vi "SLSC Create Tree Hierarchy.vi"(7 "Initialized?":bool, 8 "error in (no error)":errorcluster, 9 "SLSC EDS module":T2, 10 "Custom Device Name":string, 11 "Item Ref in":T1 format="%.0x") -> (0 "error out":errorcluster, 3 "Parent Ref out":T1 format="%.0x")   [LabVIEW 2019, in "SLSC EDS System Explorer.lvlib"]
uses:
  System Explorer/SLSC EDS System Explorer.lvlib
  SLSC EDS API/JSON parsing/EDSjsonStructure.ctl
  SLSC EDS API/JSON parsing/enum.ctl
  SLSC EDS API/JSON parsing/property.ctl
  SLSC EDS API/JSON parsing/command.ctl
  SLSC EDS API/JSON parsing/scale.ctl
  SLSC EDS API/JSON parsing/physicalChannel.ctl
  SLSC EDS API/JSON parsing/register.ctl
  <vilib>/NI VeriStand/Custom Device API/Custom Device Item Ref.ctl
  Shared/Constants.vi
  <vilib>/NI VeriStand/Custom Device API/Set Item Property (Boolean).vi
  <vilib>/NI VeriStand/Custom Device API/Set Item Property (Variant).vi
  <vilib>/NI VeriStand/Custom Device API/Set Item Property (U32).vi
  <vilib>/NI VeriStand/Custom Device API/Set Item Property (String).vi
  <vilib>/NI VeriStand/Custom Device API/Get Item Property (U32).vi
  SLSC CD System Explorer.lvlib
  <vilib>/NI VeriStand/Custom Device API/Custom Device API.lvlib
  Shared/SLSC EDS Shared.lvlib
  <vilib>/NI VeriStand/Custom Device Tools/Custom Device Utility Library/Custom Device Utility Library.lvlib
panel:
  # "not working\nregisterMap->registers->initialValue"
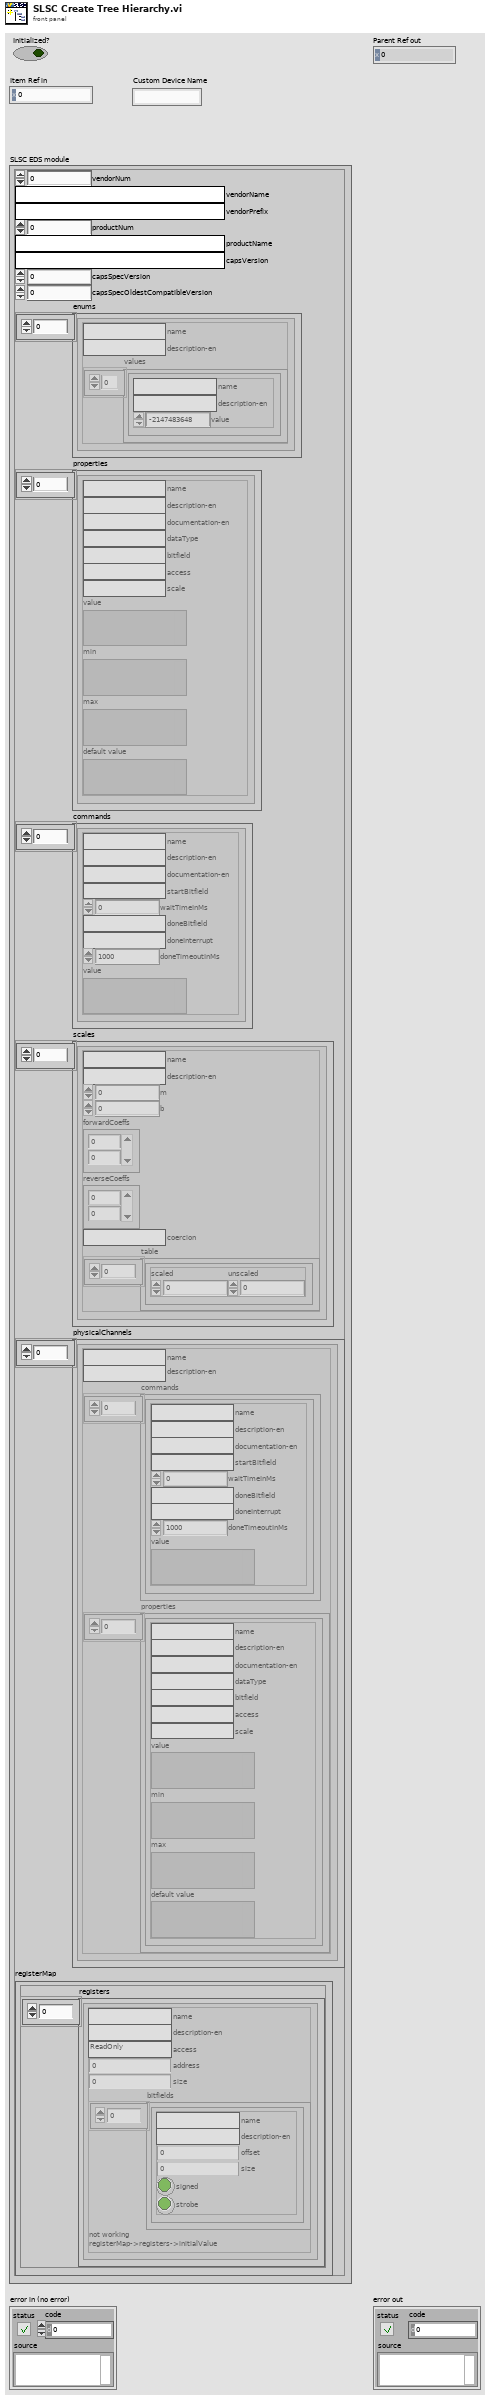
[diagram p1: front panel]
types:
  T1 = typedef "Custom Device API.lvlib/Custom Device Item Ref.ctl" = u64
  T2 = typedef "EDSjsonStructure.ctl" = cluster{"vendorNum":u32, "vendorName":string, "vendorPrefix":string, "productNum":u32, "productName":string, "capsVersion":string, "capsSpecVersion":u32, "capsSpecOldestCompatibleVersion":u32, "enums":T3[], "properties":T4[], "commands":T5[], "scales":T6[], "physicalChannels":T7[], "registerMap":cluster{"registers":T8[]}}
  T3 = typedef "enum.ctl" = cluster{"name":string, "description-en":string, "values":cluster{"name":string, "description-en":string, "value":i32}[]}
  T4 = typedef "property.ctl" = cluster{"name":string, "description-en":string, "documentation-en":string, "dataType":string, "bitfield":string, "access":string, "scale":string, "value":variant, "min":variant, "max":variant, "default value":variant}
  T5 = typedef "command.ctl" = cluster{"name":string, "description-en":string, "documentation-en":string, "startBitfield":string, "waitTimeInMs":i32, "doneBitfield":string, "doneInterrupt":string, "doneTimeoutInMs":i32, "value":variant}
  T6 = typedef "scale.ctl" = cluster{"name":string, "description-en":string, "m":dbl, "b":dbl, "forwardCoeffs":dbl[], "reverseCoeffs":dbl[], "coercion":string, "table":cluster{"scaled":dbl, "unscaled":dbl}[]}
  T7 = typedef "physicalChannel.ctl" = cluster{"name":string, "description-en":string, "commands":T5[], "properties":T4[]}
  T8 = typedef "register.ctl" = cluster{"name":string, "description-en":string, "access":string, "address":u32, "size":u32, "bitfields":cluster{"name":string, "description-en":string, "offset":u32, "size":u32, "signed":bool, "strobe":bool}[]}
  T9 = typedef "Custom Device API.lvlib/Custom Device Channel.ctl" = cluster{"Type":T10, "Units":string, "Default Value":dbl, "Faultable":bool, "Scalable":bool}
  T10 = typedef "Custom Device API.lvlib/Custom Device Channel Type.ctl" = enum16{"Input", "Output"}
  T11 = cluster{"Channel Name":string, "SLSC Name":string, "Channel":T9}[]
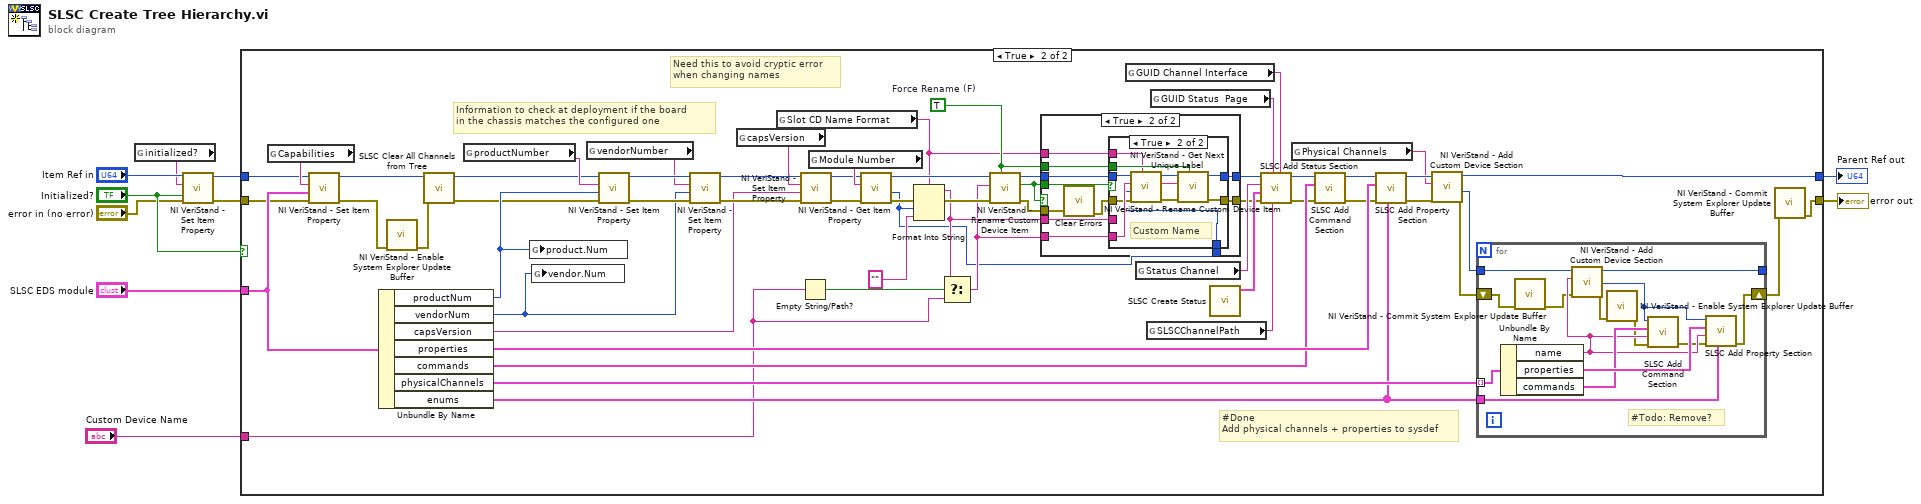
[diagram p0: block diagram]
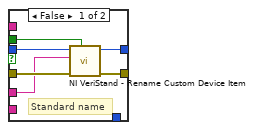
[diagram p4: hidden frame]
diagram:
  n1 = global read "Constants.vi" "initialized?"() -> (w4:string)
  n2 = call-poly <vilib>:"NI VeriStand - Set Item Property.vi"("error in (no error)"="error in (no error)", "Value"="Initialized?", "Property Name"=w4, "Item Ref in"="Item Ref in") -> ("error out"=w8:errorcluster, "Item Ref out"=w6:T1)  [unwired: 5 in, 1 out]
  n3 = case shown="True" "Initialized?" {
    tunnel: w6 -> [w12 w29]
    tunnel: "SLSC EDS module" -> [_ w63]
    tunnel: [w11 w33] -> w2
    tunnel: [w12 w47] -> w3
    tunnel: w8 -> [w11 w28]
    tunnel: "Custom Device Name" -> [_ w30]
    frame False {
    }
    frame True {
      w19 = TRUE  # Force Rename (F)
      # "Need this to avoid cryptic error \nwhen changing names"
      # "#Done\nAdd physical channels + properties to sysdef"
      # "Information to check at deployment if the board \nin the chassis matches the configured one"
      n4 = global read "Constants.vi" "Capabilities"() -> (w62:string)
      n5 = call-poly <vilib>:"NI VeriStand - Set Item Property.vi"("error in (no error)"=w28, "Value"=w63, "Property Name"=w62, "Item Ref in"=w29) -> ("error out"=w27:errorcluster, "Item Ref out"=w24:T1)  [unwired: 5 in, 1 out]
      n6 = Unbundle By Name(w63) -> ("productNum"=w46:u32, "vendorNum"=w45:u32, "capsVersion"=w67:string, "properties"=w64:T4[], "commands"=w61:T5[], "physicalChannels"=w60:T7[], "enums"=w53:T3[])
      n7 = call <vilib>:"NI VeriStand - Enable System Explorer Update Buffer.vi"("error in (no error)"=w27) -> ("error out"=w26:errorcluster)  [unwired: 10 in]
      n8 = call "SLSC Clear All Channels from Tree.vi"("error in (no error)"=w26, "Device Item Ref in"=w24) -> ("error out"=w25:errorcluster, "Item Ref out"=w23:T1)  [unwired: 8 in]
      n9 = global read "Constants.vi" "productNumber"() -> (w66:string)
      n10 = global write "Constants.vi" "product.Num"(w46) -> ()
      n11 = global write "Constants.vi" "vendor.Num"(w45) -> ()
      n12 = global read "Constants.vi" "vendorNumber"() -> (w65:string)
      n13 = call-poly <vilib>:"NI VeriStand - Set Item Property.vi"("error in (no error)"=w25, "Value"=w46, "Property Name"=w66, "Item Ref in"=w23) -> ("error out"=w69:errorcluster, "Item Ref out"=w71:T1)  [unwired: 5 in, 1 out]
      n14 = call-poly <vilib>:"NI VeriStand - Set Item Property.vi"("error in (no error)"=w69, "Value"=w45, "Property Name"=w65, "Item Ref in"=w71) -> ("error out"=w68:errorcluster, "Item Ref out"=w70:T1)  [unwired: 5 in, 1 out]
      n15 = global read "Constants.vi" "capsVersion"() -> (w52:string)
      n16 = global read "Constants.vi" "Slot CD Name Format"() -> (w16:string)
      n17 = Empty String/Path?(string/path=w30) -> (empty?=w31:bool)
      n18 = call-poly <vilib>:"NI VeriStand - Set Item Property.vi"("error in (no error)"=w68, "Value"=w67, "Property Name"=w52, "Item Ref in"=w70) -> ("error out"=w36:errorcluster, "Item Ref out"=w38:T1)  [unwired: 5 in, 1 out]
      n19 = global read "Constants.vi" "Module Number"() -> (w39:string)
      n20 = call-poly <vilib>:"NI VeriStand - Get Item Property.vi"("error in (no error)"=w36, "Property Name"=w39, "Item Ref in"=w38) -> ("error out"=w35:errorcluster, "Value"=w15:u32, "Item Ref out"=w37:T1)  [unwired: 5 in, 1 out]
      n21 = Format Into String(format string=w16, error in=w35, w15, "") -> (resulting string=w18:string, error out=w50:errorcluster)  [unwired: 1 in]
      n22 = Select(t=w18, s=w31, f=w30) -> (s? t:f=w17:string)
      n23 = call <vilib>:"NI VeriStand - Rename Custom Device Item.vi"("Force Rename (F)"=w19, "error in (no error)"=w50, "New Name"=w17, "Item Ref in"=w37) -> ("error out"=w13:errorcluster, "Request invalid?"=w14:bool, "Item Ref out"=w21:T1)  [unwired: 5 out]
      n24 = case shown="True" w14 {
        tunnel: [w72 w83] -> w22
        tunnel: w21 -> [w73 w80]
        tunnel: [w73 w79] -> w20
        tunnel: w14 -> [_ w84]
        tunnel: w19 -> [_ w82]
        tunnel: w18 -> [_ w81]
        tunnel: w17 -> [_ w78]
        tunnel: w16 -> [_ w76]
        tunnel: w15 -> [_ w75]
        tunnel: w13 -> [w72 w74]
        frame False {
        }
        frame True {
          n25 = call <vilib>:"Clear Errors.vi"("error in (no error)"=w74) -> ("error out"=w77:errorcluster)  [unwired: 5 in, 1 out]
          n26 = case shown="True" w84 {
            tunnel: w77 -> [w90 w97]
            tunnel: [w89 w101] -> w83
            tunnel: w82 -> [w88 w93]
            tunnel: w81 -> [w87 _]
            tunnel: w80 -> [w86 w100]
            tunnel: [w85 w94] -> w79
            tunnel: w78 -> [_ w98]
            tunnel: w76 -> [_ w92]
            tunnel: w75 -> [_ w91]
            frame False {
              # "Standard name"
              n27 = call <vilib>:"NI VeriStand - Rename Custom Device Item.vi"("Force Rename (F)"=w88, "error in (no error)"=w90, "New Name"=w87, "Item Ref in"=w86) -> ("error out"=w89:errorcluster, "Item Ref out"=w85:T1)  [unwired: 6 out]
            }
            frame True {
              # "Custom Name"
              n28 = call <vilib>:"NI VeriStand - Get Next Unique Label.vi"("format string"=w92, "error in (no error)"=w97, "Start Value (1)"=w91, "Label"=w98, "Parent Ref in"=w100) -> ("error out"=w96:errorcluster, "Label out"=w95:string, "Parent Ref dup"=w99:T1)  [unwired: 3 in, 1 out]
              n29 = call <vilib>:"NI VeriStand - Rename Custom Device Item.vi"("Force Rename (F)"=w93, "error in (no error)"=w96, "New Name"=w95, "Item Ref in"=w99) -> ("error out"=w101:errorcluster, "Item Ref out"=w94:T1)  [unwired: 6 out]
            }
          }
        }
      }
      n30 = global read "Constants.vi" "GUID Channel Interface"() -> (w42:string)
      n31 = global read "Constants.vi" "Status Channel"() -> (w41:string)
      n32 = global read "Constants.vi" "SLSCChannelPath"() -> (w40:string)
      n33 = global read "Constants.vi" "GUID Status  Page"() -> (w43:string)
      n34 = call "SLSC Create Status.vi"() -> ("Outgoing configuration"=w44:T11)  [unwired: 11 in]
      n35 = call "SLSC Add Status Section.vi"("GUID Channel Interface"=w42, "SLSC Channel Path"=w40, "GUID (Default Section)"=w43, "error in (no error)"=w22, "Outgoing configuration"=w44, "Section Name"=w41, "Parent Ref in"=w20) -> ("error out"=w48:errorcluster, "Parent Ref out"=w49:T1)  [unwired: 3 in]
      n36 = global read "Constants.vi" "Physical Channels"() -> (w51:string)
      n37 = call "SLSC Add Command Section.vi"("error in (no error)"=w48, "commands"=w61, "Parent Ref in"=w49) -> ("error out"=w55:errorcluster, "Parent Ref out"=w59:T1)  [unwired: 7 in]
      n38 = call "SLSC Add Property Section.vi"("enums"=w53, "error in (no error)"=w55, "properties"=w64, "Parent Ref in"=w59) -> ("error out"=w54:errorcluster, "Parent Ref out"=w58:T1)  [unwired: 6 in]
      n39 = call <vilib>:"NI VeriStand - Add Custom Device Section.vi"("error in (no error)"=w54, "Section Name"=w51, "Parent Ref in"=w58) -> ("error out"=w56:errorcluster, "Section Ptr"=w57:T1, "Parent Ref out"=w47:T1)  [unwired: 5 in, 1 out]
      n40 = for {
        tunnel: w60 -> [w115] mode=indexing
        shift-right: [w104] -> w34
        shift-left: w56 -> [w106]
        tunnel: w57 -> [w112]
        tunnel: [w111] -> _
        tunnel: w53 -> [w108]
        # "#Todo: Remove?"
        n41 = Unbundle By Name(w115) -> ("name"=w110:string, "properties"=w114:T4[], "commands"=w113:T5[])
        n42 = call <vilib>:"NI VeriStand - Commit System Explorer Update Buffer.vi"("error in (no error)"=w106) -> ("error out"=w105:errorcluster)  [unwired: 10 in]
        n43 = call <vilib>:"NI VeriStand - Add Custom Device Section.vi"("error in (no error)"=w105, "Section Name"=w110, "Parent Ref in"=w112) -> ("error out"=w103:errorcluster, "Section Ptr"=w107:T1, "Parent Ref out"=w111:T1)  [unwired: 5 in, 1 out]
        n44 = call <vilib>:"NI VeriStand - Enable System Explorer Update Buffer.vi"("error in (no error)"=w103) -> ("error out"=w102:errorcluster)  [unwired: 10 in]
        n45 = call "SLSC Add Command Section.vi"("error in (no error)"=w102, "Physical Channel"=w110, "commands"=w113, "Parent Ref in"=w107) -> ("error out"=w109:errorcluster)  [unwired: 6 in, 1 out]
        n46 = call "SLSC Add Property Section.vi"("enums"=w108, "error in (no error)"=w109, "Physical Channel"=w110, "properties"=w114, "Parent Ref in"=w107) -> ("error out"=w104:errorcluster)  [unwired: 5 in, 1 out]
      }
      n47 = call <vilib>:"NI VeriStand - Commit System Explorer Update Buffer.vi"("error in (no error)"=w34) -> ("error out"=w33:errorcluster)  [unwired: 10 in]
    }
  }
  "Parent Ref out" <- w3
  "error out" <- w2
